vi "Weather Station UI.vi"() -> ()   [LabVIEW 2014]
doc: "本VI是气象站项目的主VI。其中包含用于温度警告系统的用户界面。每间隔半秒读取温度；发生警告时记录数据。"
uses:
  Supporting Files/Weather Station States.ctl
  Supporting Files/Weather Data.ctl
  Instance           2 26Saved   Weather Station UI .vi
panel:
  out "警告":string
  in  "下限":dbl=20.0
  in  "上限":dbl=30.0
  in  "停止按钮":bool
  out "温度历史":dbl(graph)
  # "温度范围 (C)"
  # "冷冻"
  # "中暑"
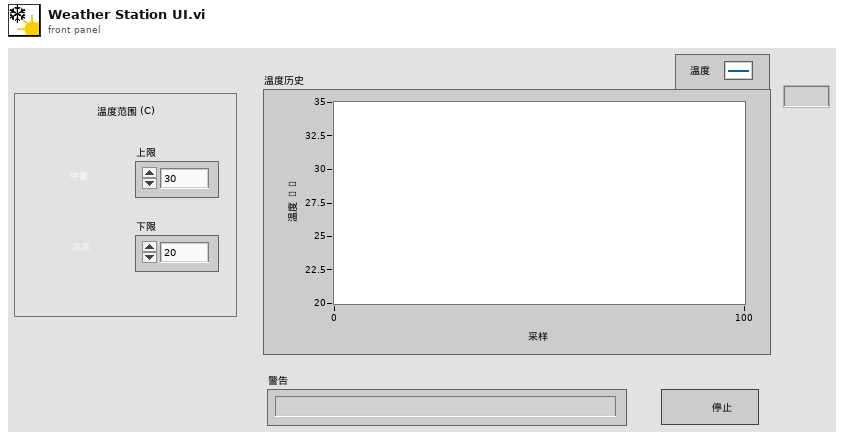
[diagram p1: front panel]
types:
  T1 = enum16{"open", "replace", "create", "open or create", "replace or create", "replace or create with confirmation"}
  T2 = typedef "Weather Data.ctl" = cluster{"当前温度":dbl, "最高温度":dbl, "最低温度":dbl, "温度警告？":bool, "温度警告文本":string}
  T3 = typedef "Weather Station States.ctl" = enum16{"采集", "分析", "数据记录", "时间检查"}
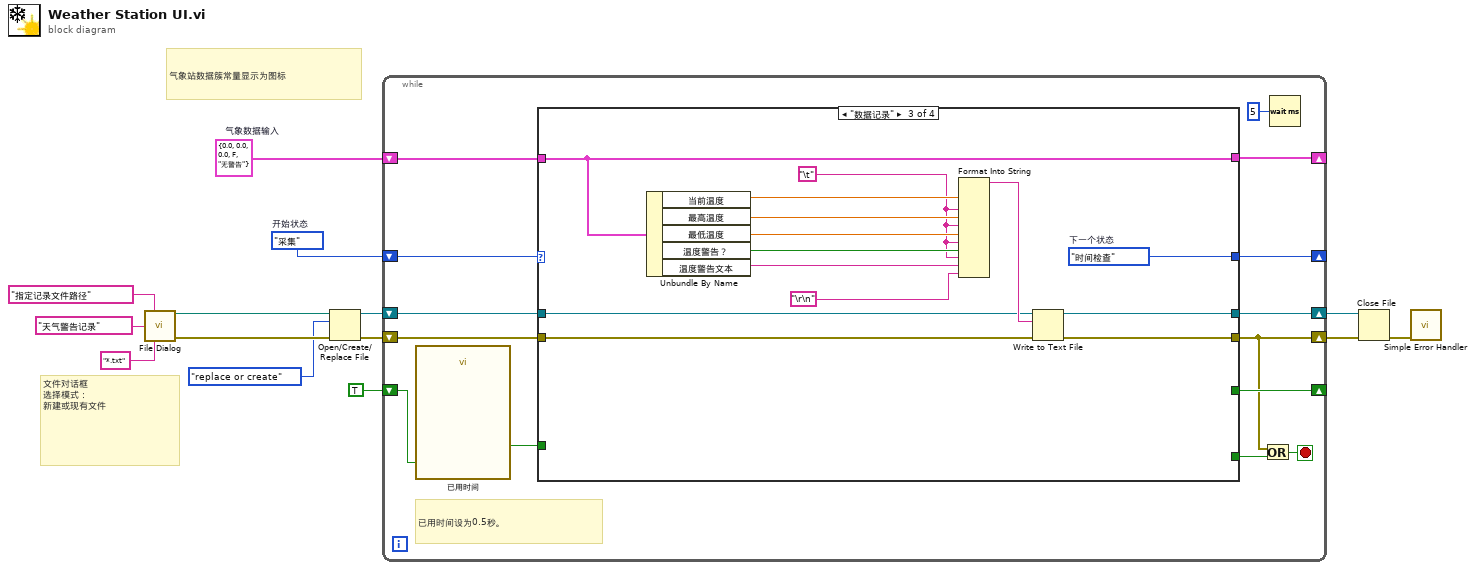
[diagram p0: block diagram]
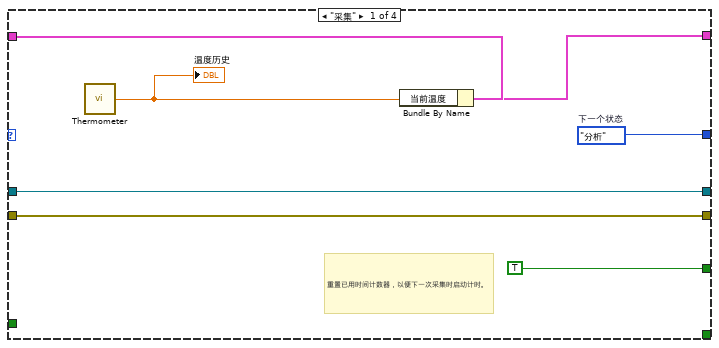
[diagram p2: hidden frame]
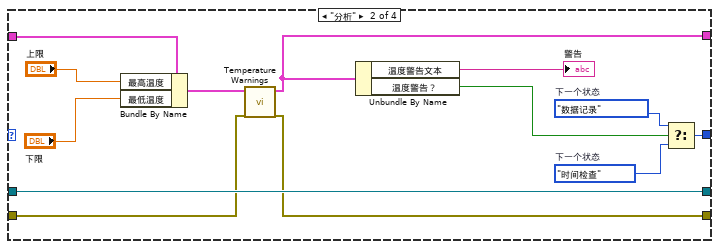
[diagram p3: hidden frame]
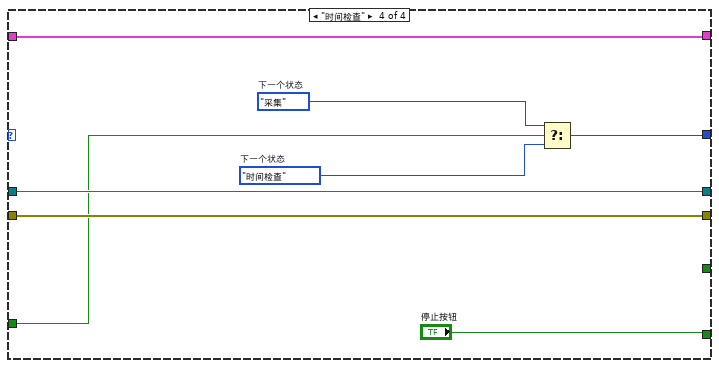
[diagram p4: hidden frame]
diagram:
  w7 = T2 {"当前温度"=0.0, "最高温度"=0.0, "最低温度"=0.0, "温度警告？"=FALSE, "温度警告文本"="无警告"}  # 气象数据输入
  w14 = Weather_Station_States."采集"  # 开始状态
  # "文件对话框\n选择模式：\n新建或现有文件"
  # "气象站数据簇常量显示为图标"
  n1 = call "File Dialog"("prompt"="指定记录文件路径" ("提示"), "default name"="天气警告记录" ("默认名称"), "pattern (all files)"="*.txt" ("类型标签")) -> ("selected path"=w6:path, "error out"=w3:errorcluster)  [unwired: 9 in, 2 out]
  n2 = Open/Create/Replace File(file path (use dialog)=w6, error in=w3, operation (0:open)=T1."replace or create" ("操作(0:open)")) -> (refnum out=w9:refnum<file>, error out=w8:errorcluster)  [unwired: 3 in, 1 out]
  n3 = while {
    shift-right: [w27] -> _
    shift-left: w14 -> [w28]
    shift-right: [w15] -> w13
    shift-left: w8 -> [w26]
    shift-right: [w16] -> _
    shift-left: w7 -> [w23]
    shift-right: [w24] -> w12
    shift-left: w9 -> [w22]
    shift-right: [w17] -> _
    shift-left: TRUE ("停止") -> [w19]
    stop <- w25 stop-if-true
    # "已用时间设为0.5秒。"
    n4 = call "已用时间"("Reset"=w19) -> ("Time has Elapsed"=w18:bool)  [unwired: 11 in, 7 out]
    n5 = case shown="\"数据记录\"" w28 {
      tunnel: [w35 w42 w62 w63] -> w27
      tunnel: [w30 w46 w60 w69] -> w15
      tunnel: w26 -> [w30 w47 w61 w69]
      tunnel: [w34 w48 w59 w70] -> w24
      tunnel: [w31 w41 w51 w68] -> w16
      tunnel: w23 -> [w32 w39 w51 w68]
      tunnel: w22 -> [w34 w48 w57 w70]
      tunnel: [_ _ _ "停止按钮"] -> w21
      tunnel: w18 -> [_ _ _ w64]
      tunnel: [TRUE ("停止") _ _ _] -> w17
      frame "采集" {
        w35 = Weather_Station_States."分析"  # 下一个状态
        # "重置已用时间计数器，以便下一次采集时启动计时。"
        n6 = call "Thermometer.vi"() -> ("温度"=w29:dbl)  [unwired: 1 in]
        "温度历史" <- w29
        n7 = Bundle By Name(cluster=w32, "当前温度"=w29) -> (w31:T2)
      }
      frame "分析" {
        w44 = Weather_Station_States."数据记录"  # 下一个状态
        w43 = Weather_Station_States."时间检查"  # 下一个状态
        n8 = Bundle By Name(cluster=w39, "最高温度"="上限", "最低温度"="下限") -> (w38:T2)
        n9 = call "Temperature Warnings.vi"("错误输入"=w47, "气象数据输入"=w38) -> ("错误输出"=w46:cluster{"状态":bool, "代码":i32, "源":string}, "气象数据输出"=w41:T2)  [unwired: 8 in]
        n10 = Unbundle By Name(w41) -> ("温度警告文本"=→"警告":string, "温度警告？"=w45:bool)
        n11 = Select(t=w44, s=w45, f=w43) -> (s? t:f=w42:T3)
      }
      frame "数据记录" {
        w62 = Weather_Station_States."时间检查"  # 下一个状态
        w50 = "\t" ("制表符常量")
        n12 = Unbundle By Name(w51) -> ("当前温度"=w56:dbl, "最高温度"=w55:dbl, "最低温度"=w54:dbl, "温度警告？"=w53:bool, "温度警告文本"=w49:string)
        n13 = Format Into String(w56, w50, w55, w50, w54, w50, w53, w50, w49, "\r\n" ("行结束常量")) -> (resulting string=w58:string)  [unwired: 3 in, 1 out]
        n14 = Write to Text File(file (use dialog)=w57, text=w58, error in=w61) -> (refnum out=w59:refnum<file>, error out=w60:errorcluster)  [unwired: 1 in, 1 out]
      }
      frame "时间检查" {
        w66 = Weather_Station_States."时间检查"  # 下一个状态
        w65 = Weather_Station_States."采集"  # 下一个状态
        n15 = Select(t=w65, s=w64, f=w66) -> (s? t:f=w63:T3)
      }
    }
    n16 = Or(x=w15, y=w21) -> (x .or. y?=w25:bool)
    n17 = Wait (ms)(milliseconds to wait=u32 5 ("y")) -> ()  [unwired: 1 out]
  }
  n18 = Close File(refnum=w12, error in=w13) -> (error out=w11:errorcluster)  [unwired: 1 out]
  n19 = call <vilib>:"Simple Error Handler.vi"("error in (no error)"=w11) -> ()  [unwired: 4 in, 5 out]
